vi "deletePPMS.GET ALL.vi"(8 "error in (no error)":errorcluster, 11 "instrument.PPMS":refnum<class "instrument.PPMS.lvclass">) -> (0 "error out":errorcluster, 2 "getAll":T1, 3 "instrument.PPMS out":refnum<class "instrument.PPMS.lvclass">)   [LabVIEW 2019]
uses:
  51190d81-5331-44c5-ae51-655eeb647297.vi
  Typedefs/PPMS.getAll--cluster.ctl
  instrument.PPMS.lvclass
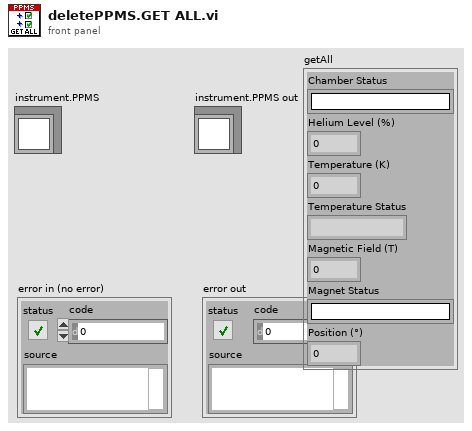
[diagram p1: front panel]
types:
  T1 = typedef "instrument.PPMS.lvclass/PPMS.getAll--cluster.ctl" = cluster{"Chamber Status":string, "Helium Level (%)":dbl, "Temperature (K)":dbl, "Temperature Status":string, "Magnetic Field (T)":dbl, "Magnet Status":string, "Position (°)":dbl}
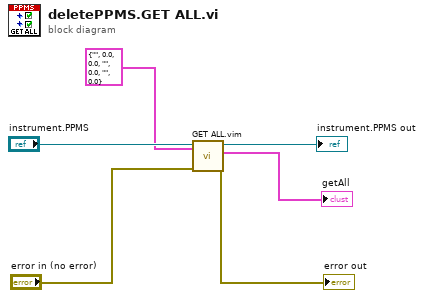
[diagram p0: block diagram]
diagram:
  n1 = call "GET ALL.vim"("type"=T1 {"Chamber Status"="", "Helium Level (%)"=0.0, "Temperature (K)"=0.0, "Temperature Status"="", "Magnetic Field (T)"=0.0, "Magnet Status"="", "Position (°)"=0.0} ("getAll"), "error in (no error)"="error in (no error)", "Instrument in"="instrument.PPMS") -> ("error out"=→"error out":errorcluster, "getAll"=→"getAll":T1, "Instrument out"=→"instrument.PPMS out":refnum<class "instrument.PPMS.lvclass">)  [unwired: 6 in]
